vi "Set_Mono.vi"(8 "error in (no error)":errorcluster, 10 "Mono On":bool, 11 "NKT in":refnum<class "NKT_Extreme.lvclass">) -> (0 "error out":errorcluster, 3 "NKT out":refnum<class "NKT_Extreme.lvclass">)   [LabVIEW 2020, in "NKT_Extreme.lvclass"]
uses:
  <instrlib>/Classes/Laser/NKT/NKT_Extreme.lvclass
  <instrlib>/NKTP_API/NKTP_API.lvlib
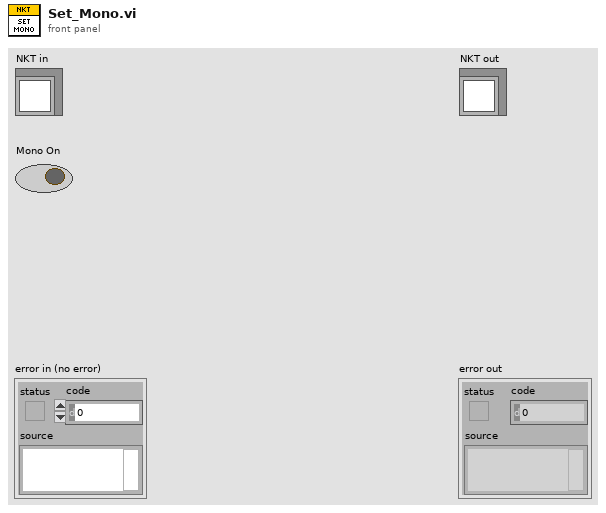
[diagram p1: front panel]
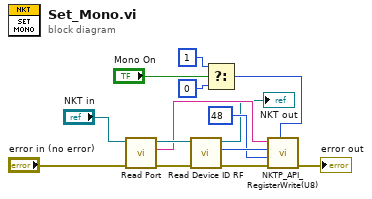
[diagram p0: block diagram]
diagram:
  n1 = call-dynamic "Read Port.vi"("error in (no error)"="error in (no error)", "NKT in"="NKT in") -> ("error out"=w12:errorcluster, "Port"=w10:string, "NKT out"=w11:refnum<class "NKT_Extreme.lvclass">)  [unwired: 7 in]
  n2 = call-dynamic "Read Device ID RF.vi"("error in (no error)"=w12, "NKT in"=w11) -> ("error out"=w6:errorcluster, "Device ID RF"=w9:u8, "NKT out"=→"NKT out":refnum<class "NKT_Extreme.lvclass">)  [unwired: 7 in]
  n3 = Select(t=u8 1 ("regId"), s="Mono On", f=u8 0 ("regId")) -> (s? t:f=w1:u8)
  n4 = call <instrlib>:"NKTP_API_RegisterWrite(U8).vi"("value"=w1, "error in"=w6, "regId"=u8 48, "devId"=w9, "portname"=w10) -> ("error out"=→"error out":errorcluster)  [unwired: 5 in, 1 out]
